vi "ATPassthru.vi"(10 "read buffer":string, 11 "VISA Refnum in":refnum<visa-resource-name>) -> ()   [LabVIEW 2014, in "Acquisition.lvlib"]
uses:
  <vilib>/Instr/_visa.llb/VISA Configure Serial Port (Instr).vi
  Acquisition.lvlib
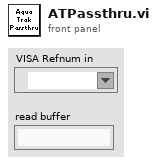
[diagram p1: front panel]
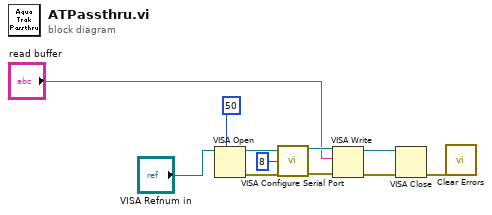
[diagram p0: block diagram]
diagram:
  n1 = VISA Open(timeout (0)=u32 50 ("VISA Open timeout (0)"), VISA resource name="VISA Refnum in") -> (VISA resource name=w5:refnum<visa-resource-name>, error out=w6:errorcluster)  [unwired: 3 in]
  n2 = call-poly "VISA Configure Serial Port"("VISA resource name"=w5, "data bits (8)"=u16 8, "error in (no error)"=w6) -> ("VISA resource name out"=w7:refnum<visa-resource-name>, "error out"=w8:errorcluster)  [unwired: 11 in]
  n3 = VISA Write(VISA resource name=w7, write buffer="read buffer", error in (no error)=w8) -> (VISA resource name out=w3:refnum<visa-resource-name>, error out=w2:errorcluster)  [unwired: 1 out]
  n4 = VISA Close(VISA resource name=w3, error in (no error)=w2) -> (error out=w11:errorcluster)
  n5 = call <vilib>:"Clear Errors.vi"("error in (no error)"=w11) -> ()  [unwired: 5 in, 2 out]
